vi "Log One-Second Interval Message (if necessary).vi"(8 "Error In":errorcluster, 11 "Errors in current one-second interval":T1[](array[typedef])) -> (0 "Error Out":errorcluster)   [LabVIEW 2023, in "Error Manager.lvlib"]
doc: "Blank VI with error handling."
uses:
  Error Manager.lvlib
  Error in current one-second interval (cluster).ctl
panel:
  # "Input\nInputs to the VI"
  # "Development\nControls or indicators that are useful for development or testing, but which are not outputs of the VI."
  # "Output\nOutputs of the VI"
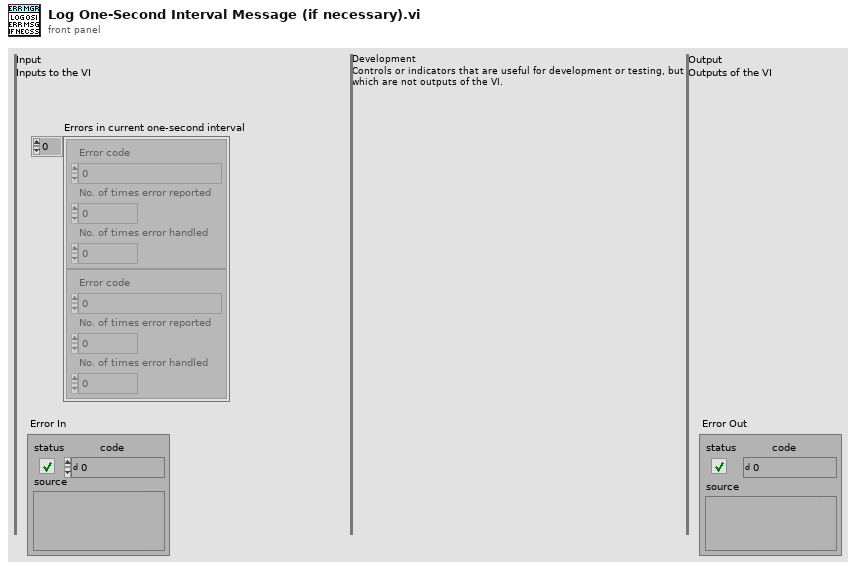
[diagram p1: front panel]
types:
  T1 = typedef "Error Manager.lvlib/Error in current one-second interval (cluster).ctl" = cluster{"Error code":i32, "No. of times error reported":u32, "No. of times error handled":u32}
  T2 = typedef "Error Manager.lvlib/Unhandled Error (cluster).ctl" = cluster{"Error code":i32, "No. of times error reported but not handled":u32}
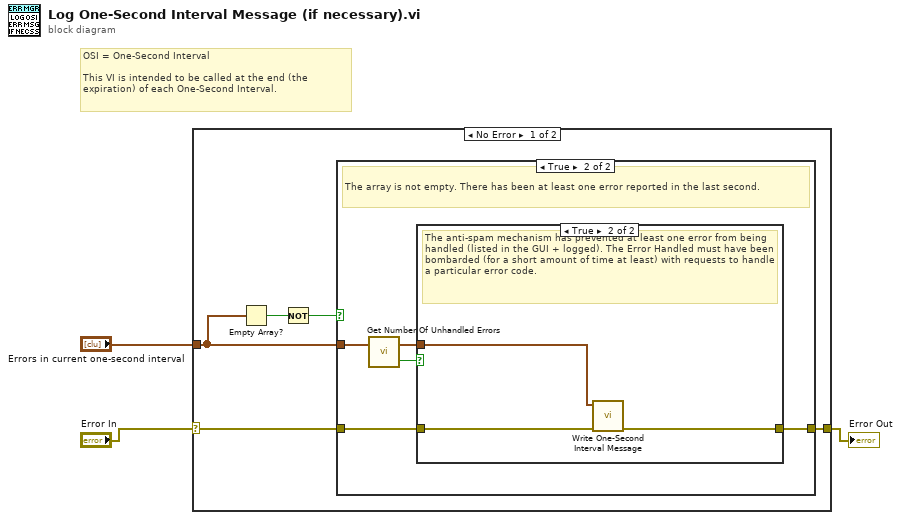
[diagram p0: block diagram]
diagram:
  # "OSI = One-Second Interval\n\nThis VI is intended to be called at the end (the expiration) of each One-Second Interval."
  n1 = case shown="No Error" "Error In" {
    selector: "Error In" -> [w8 w19]
    tunnel: [w7 w19] -> w2
    tunnel: "Errors in current one-second interval" -> [w4 _]
    frame No Error {
      n2 = Empty Array?(array=w4) -> (empty?=w6:bool)
      n3 = Not(x=w6) -> (.not. x?=w5:bool)
      n4 = case shown="True" w5 {
        tunnel: w8 -> [w9 w14]
        tunnel: [w9 w13] -> w7
        tunnel: w4 -> [_ w12]
        frame False {
          # "Do nothing. No extra message to write to erro log."
          # "The OSI data structure is empty. This means no new errors whatsoever were reported to the error handler module in the last second. This is ok and expected to execute most of the time."
        }
        frame True {
          # "The array is not empty. There has been at least one error reported in the last second."
          n5 = call "Get Number Of Unhandled Errors.vi"(3:w12) -> (0:w11:bool, 1:w10:T2[])  [unwired: 1 in]
          n6 = case shown="True" w11 {
            tunnel: w14 -> [w15 w18]
            tunnel: [w15 w17] -> w13
            tunnel: w10 -> [_ w16]
            frame False {
              # "There are no unhandled errors. The Error Handler module has not been bombarded with 'Handle Error' requests. This case expected to execute most of the time."
            }
            frame True {
              # "The anti-spam mechanism has prevented at least one error from being handled (listed in the GUI + logged). The Error Handled must have been bombarded (for a short amount of time at least) with requests to handle a particular error code."
              n7 = call "Write One-Second Interval Message.vi"(8:w18, 11:w16) -> (0:w17:errorcluster)  [unwired: 9 in]
            }
          }
        }
      }
    }
    frame Error {
    }
  }
  "Error Out" <- w2
